vi "Camera_PhotonFocus.vi"() -> ()   [LabVIEW 2012]
uses:
  <vilib>/userdefined/High Color/IMAQdx.ctl
  <vilib>/vision/driver/NI_Vision_Acquisition_Software.lvlib
  <resource>/objmgr/imaqdx.rc
panel:
  out "all stop":bool
  in  "stop":bool
  in  "reset exposure":bool
  in  "Exposure \nTime (ms)":dbl=200.0
  out "Image":T1(plugin-control)
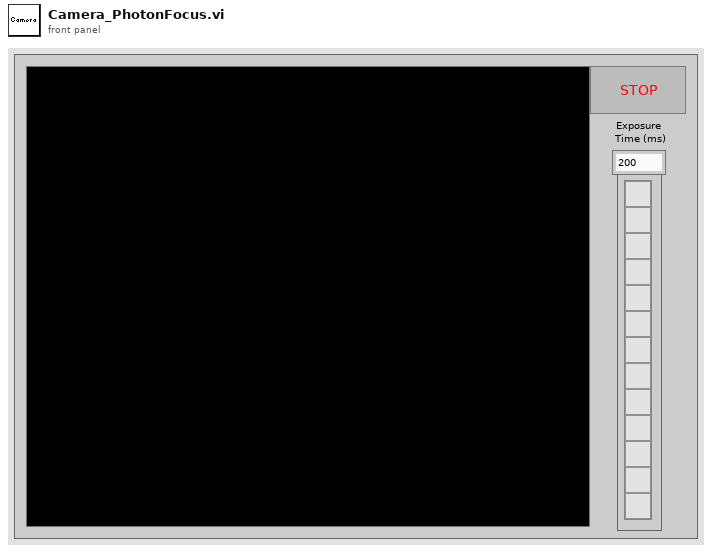
[diagram p1: front panel]
types:
  T1 = typedef "IMAQ Image.ctl" = refnum<image>
  T2 = typedef "IMAQdx.ctl" = refnum<k21>
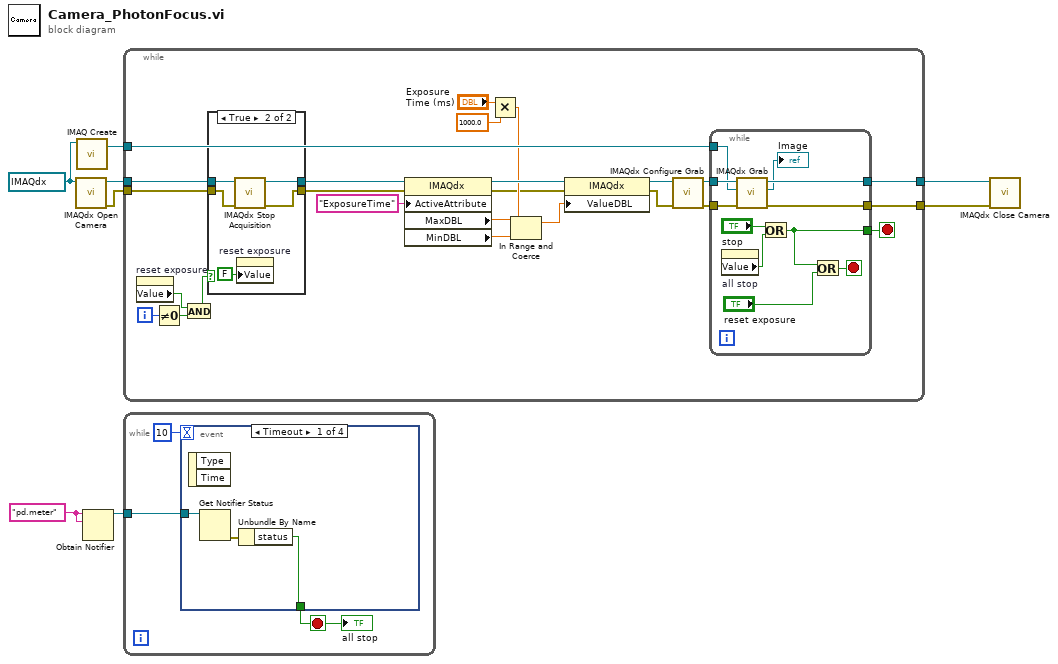
[diagram p0: block diagram]
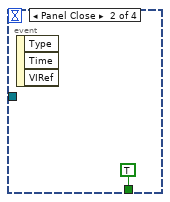
[diagram p2: hidden frame]
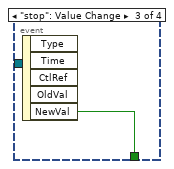
[diagram p3: hidden frame]
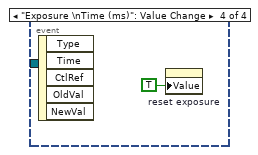
[diagram p4: hidden frame]
diagram:
  w2 = "pd.meter" ("Tag in")
  w8 = T2 "cam0" ("Session In")
  n1 = call <vilib>:"IMAQdx Open Camera.vi"("Session In"=w8) -> ("error out"=w3:errorcluster, "Session Out"=w7:T2)  [unwired: 9 in]
  n2 = call "IMAQ Create"("Image Name"=w8) -> ("New Image"=w6:T1)  [unwired: 4 in, 1 out]
  n3 = Obtain Notifier(name (unnamed)=w2, notification data type=w2) -> (notifier out=w1:refnum<notifier>)  [unwired: 2 in, 2 out]
  n4 = while {
    tunnel: w7 -> [w16]
    tunnel: w6 -> [w31]
    tunnel: [w30] -> w5
    tunnel: [w29] -> w4
    tunnel: w3 -> [w14]
    i -> [w12]
    stop <- w17 stop-if-true
    n5 = property on="reset exposure" class="Bool (strict)"() -> ("Value"=w10:bool)  [unwired: 2 in, 2 out]
    n6 = Not Equal To 0?(x=w12) -> (x != 0?=w11:bool)
    n7 = And(x=w10, y=w11) -> (x .and. y?=w9:bool)
    n8 = case shown="True" w9 {
      tunnel: [w35 w37] -> w15
      tunnel: w16 -> [w35 w40]
      tunnel: w14 -> [w34 w39]
      tunnel: [w34 w38] -> w13
      frame False {
      }
      frame True {
        n9 = call <vilib>:"IMAQdx Stop Acquisition.vi"("error in"=w39, "Session In"=w40) -> ("error out"=w38:errorcluster, "Session Out"=w37:T2)  [unwired: 8 in]
        n10 = property on="reset exposure" class="Bool (strict)"("Value"=FALSE ("reset exposure")) -> ()  [unwired: 2 in, 2 out]
      }
    }
    n11 = property class="IMAQdx"(reference=w15, error in=w13, "ActiveAttribute"="ExposureTime") -> (reference out=w28:T2, error out=w20:errorcluster, "MaxDBL"=w25:dbl, "MinDBL"=w26:dbl)
    n12 = Multiply(x="Exposure \nTime (ms)", y=1000.0) -> (x*y=w23:dbl)
    n13 = In Range and Coerce(upper limit=w25, x=w23, lower limit=w26) -> (coerced(x)=w19:dbl)  [unwired: 1 out]
    n14 = property class="IMAQdx"(reference=w28, error in=w20, "ValueDBL"=w19) -> (reference out=w21:T2, error out=w18:errorcluster)
    n15 = call <vilib>:"IMAQdx Configure Grab.vi"("error in"=w18, "Session In"=w21) -> ("error out"=w32:errorcluster, "Session Out"=w33:T2)  [unwired: 8 in]
    n16 = while {
      tunnel: w33 -> [w50]
      tunnel: w32 -> [w51]
      tunnel: w31 -> [w49]
      tunnel: [w48] -> w30
      tunnel: [w47] -> w29
      tunnel: [w42] -> w17
      stop <- w41 stop-if-true
      n17 = property on="all stop" class="Bool (strict)"() -> ("Value"=w44:bool)  [unwired: 2 in, 2 out]
      n18 = call <vilib>:"IMAQdx Grab.vi"("error in"=w51, "Image In"=w49, "Session In"=w50) -> ("error out"=w47:errorcluster, "Image Out"=→"Image":T1, "Session Out"=w48:T2)  [unwired: 5 in, 1 out]
      n19 = Or(x="stop", y=w44) -> (x .or. y?=w42:bool)
      n20 = Or(x=w42, y="reset exposure") -> (x .or. y?=w41:bool)
    }
  }
  n21 = while {
    tunnel: w1 -> [w53]
    stop <- w52 stop-if-true
    n22 = event shown="[0] Timeout" {
      selector: _ -> [_ _ _ _]
      dyn-events: _ -> [_ _ _ _]
      timeout: 10 -> [_ _ _ _]
      tunnel: [w57 TRUE ("NewVal") w59 _] -> w52
      tunnel: w53 -> [w56 _ _ _]
      event Timeout {
        n23 = event-data() -> ()  [unwired: 1 in, 2 out]
        n24 = Get Notifier Status(notifier=w56) -> (error out=w55:errorcluster)  [unwired: 1 in, 4 out]
        n25 = Unbundle By Name(w55) -> ("status"=w57:bool)
      }
      event Panel Close {
        n26 = event-data() -> ()  [unwired: 1 in, 3 out]
      }
      event "stop": Value Change {
        n27 = event-data() -> ("NewVal"=w59:bool)  [unwired: 1 in, 4 out]
      }
      event "Exposure \nTime (ms)": Value Change {
        n28 = event-data() -> ()  [unwired: 1 in, 5 out]
        n29 = property on="reset exposure" class="Bool (strict)"("Value"=TRUE ("reset exposure")) -> ()  [unwired: 2 in, 2 out]
      }
    }
    "all stop" <- w52
  }
  n30 = call <vilib>:"IMAQdx Close Camera.vi"("error in"=w4, "Session In"=w5) -> ()  [unwired: 9 in, 1 out]
